vi "Configure Duty Cycle.vi"(7 "Channel (1:Chan A)":i32(ring)=1 items=["System (To)", "Channel A", "Channel B", "Channel C", "Channel D", "Channel E", "Channel F", "Channel G", "Channel H"], 8 "error in (no error)":errorcluster, 9 "DC Off (10)":i32=10, 10 "DC On (10)":i32=10, 11 "VISA resource name":refnum<visa-resource-name>) -> (0 "error out":errorcluster, 3 "VISA resource name out":refnum<visa-resource-name>)   [LabVIEW 2012, in "Quantum Composers 9000 Series.lvlib"]
doc: "This VI is used to configure the Duty Cycle mode of operation for the selected channel or the system timer (To)."
uses:
  Quantum Composers 9000 Series.lvlib
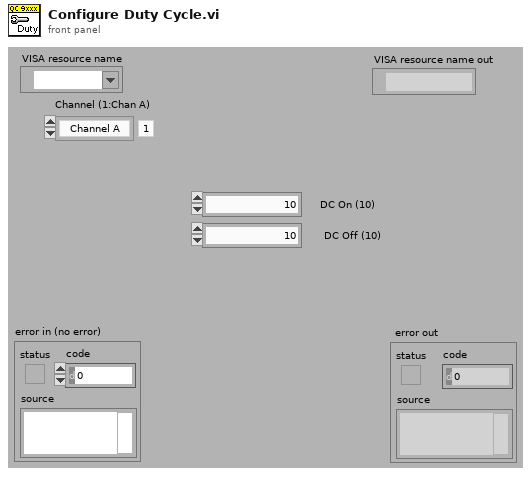
[diagram p1: front panel]
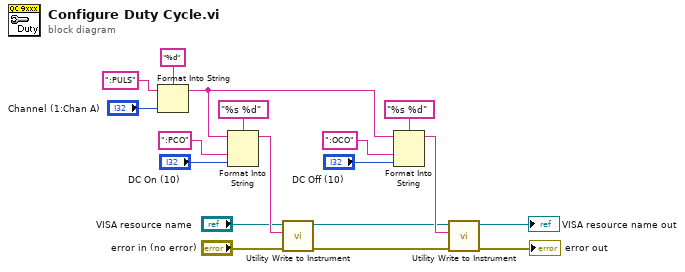
[diagram p0: block diagram]
diagram:
  n1 = Format Into String(format string="%d", initial string=":PULS", "Channel (1:Chan A)") -> (resulting string=w1:string)  [unwired: 1 in, 1 out]
  n2 = Format Into String(format string="%s %d", initial string=w1, ":PCO", "DC On (10)") -> (resulting string=w12:string)  [unwired: 1 in, 1 out]
  n3 = call "Utility Write to Instrument.vi"("error in (no error)"="error in (no error)", "Write Buffer"=w12, "VISA resource name"="VISA resource name") -> ("error out"=w7:errorcluster, "VISA resource name out"=w8:refnum<visa-resource-name>)  [unwired: 6 in, 1 out]
  n4 = Format Into String(format string="%s %d", initial string=w1, ":OCO", "DC Off (10)") -> (resulting string=w11:string)  [unwired: 1 in, 1 out]
  n5 = call "Utility Write to Instrument.vi"("error in (no error)"=w7, "Write Buffer"=w11, "VISA resource name"=w8) -> ("error out"=→"error out":errorcluster, "VISA resource name out"=→"VISA resource name out":refnum<visa-resource-name>)  [unwired: 6 in, 1 out]
